vi "Turn to Heading Calibrations.vi"() -> ()   [LabVIEW 2016]
panel:
  out "Turn to Heading Derivative Gain":dbl
  out "Turn to Heading Integral Gain":dbl
  out "Turn to Heading Proportional Gain":dbl
  out "Right Turn to Heading Derivative Gain":dbl
  out "Right Turn to Heading Feed-Forward Gain":dbl
  out "Right Turn to Heading Proportional Gain":dbl
  out "Right Turn to Heading Integral Gain":dbl
  out "Left Turn to Heading Derivative Gain":dbl
  out "Left Turn to Heading Feed-Forward Gain":dbl
  out "Left Turn to Heading Proportional Gain":dbl
  out "Left Turn to Heading Integral Gain":dbl
  in  "Turn to Heading Calibrations File Location":path=path "C:/ni-rt/startup/TurnToHeadingCalibrations.txt"
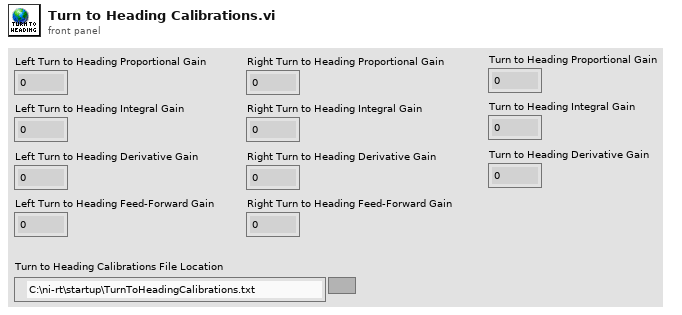
[diagram p1: front panel]
diagram:
